vi "relay_read.vi"(2 "relay session in":T1={"VISA resource out"="COM12", "error out"={"status"=FALSE, "code"=0, "source"=""}}) -> (4 "Stop Gas Flow":bool, 5 "relay session out":T1={"VISA resource out"="COM12", "error out"={"status"=FALSE, "code"=0, "source"=""}}, 6 "Dump":bool, 7 "Acid Pump":bool, 8 "Airflush":bool)   [LabVIEW 2010]
panel:
  out "code message":dbl
  out "bytes read":dbl
  out "string message":string
  # "NOTE: The relay device does not take kindly to having more bytes read from port than it actually has there. Meanwhile, LabVIEW likes to warn you when you only read as many bytes as are at the port. Living with LabVIEW warnings trumps relay errors, so that is what we went with."
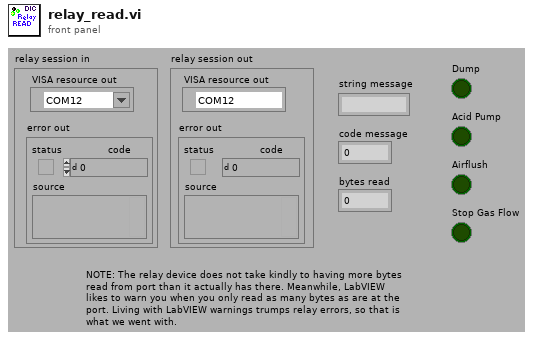
[diagram p1: front panel]
types:
  T1 = cluster{"VISA resource out":refnum<visa-resource-name>, "error out":errorcluster}
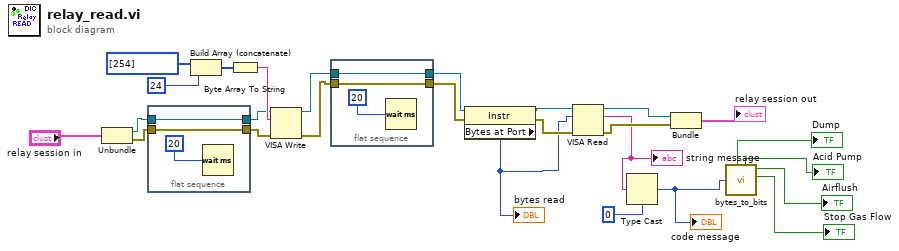
[diagram p0: block diagram]
diagram:
  n1 = Unbundle("relay session in") -> ("VISA resource out"=w5:refnum<visa-resource-name>, "error out"=w4:errorcluster)
  n2 = flat-sequence {
    tunnel: w5 -> [w29]
    tunnel: w4 -> [w28]
    tunnel: [w29] -> w2
    tunnel: [w28] -> w3
    frame #0 {
      n3 = Wait (ms)(milliseconds to wait=20) -> ()  [unwired: 1 out]
    }
  }
  n4 = Build Array (concatenate)(u8[] [254] ("unsigned byte array"), 24) -> (w24:i32[])
  n5 = Byte Array To String(unsigned byte array=w24) -> (string=w26:string)
  n6 = VISA Write(VISA resource name=w2, write buffer=w26, error in (no error)=w3) -> (VISA resource name out=w16:refnum<visa-resource-name>, error out=w15:errorcluster)  [unwired: 1 out]
  n7 = flat-sequence {
    tunnel: w16 -> [w32]
    tunnel: w15 -> [w31]
    tunnel: [w32] -> w14
    tunnel: [w31] -> w13
    frame #0 {
      n8 = Wait (ms)(milliseconds to wait=20) -> ()  [unwired: 1 out]
    }
  }
  n9 = property class="Instr"(reference=w14, error in=w13) -> (reference out=w20:refnum<visa-resource-name>, error out=w19:errorcluster, "Bytes at Port"=w1:u32)
  "bytes read" <- w1
  n10 = VISA Read(VISA resource name=w20, byte count=w1, error in (no error)=w19) -> (VISA resource name out=w18:refnum<visa-resource-name>, read buffer=w12:string, error out=w17:errorcluster)  [unwired: 1 out]
  "string message" <- w12
  n11 = Type Cast(type=i8 0, x=w12) -> (*(type *) &x=w10:i8)
  "code message" <- w10
  n12 = Bundle("VISA resource out"=w18, "error out"=w17) -> (→"relay session out":T1)  [unwired: 1 in]
  n13 = call "bytes_to_bits.vi"("Numeric"=w10) -> ("bit 1"=→"Dump":bool, "bit 2"=→"Acid Pump":bool, "bit 3"=→"Airflush":bool, "bit 4"=→"Stop Gas Flow":bool)  [unwired: 2 in, 4 out]
